vi "Get All Process Names.vi"(11 "?":T9 {"Main Config"."PR Module Configs"."Settings"."PID 2 Parameters"."output range"."output low" format="%.2f"; "Main Config"."PR Module Configs"."Settings"."PID 2 Parameters"."output range"."output high" min=0.0 max=100.0 format="%.2f"; "Main Config"."PR Module Configs"."Settings"."PID 2 Parameters"."PID gains"."derivative time (Td, min)" format="%.3f"; "Main Config"."PR Module Configs"."Settings"."PID 2 Parameters"."PID gains"."integral time (Ti, min)" format="%.3f"; "Main Config"."PR Module Configs"."Settings"."PID 2 Parameters"."PID gains"."proportional gain (Kc)" format="%.3f"; "Main Config"."Steps"."Control" items=["Pump %", "Setpoint"]; "Main Config"."TCU Module Configs"."Settings"."Huber Unistat 410 Settings"."Address" min=0 max=99 format="%02.0f"; "Main Config"."TCU Module Configs"."Settings"."Julabo FP-50 Settings"."Pump Power" min=0 max=8 step=1; "Main Config"."TCU Module Configs"."Settings"."Lauda Settings"."Pump Power" min=0 max=8 step=1; "Main Config"."Pump Module Configs"."Settings"."ASIA Pump C"."channel" min=0 max=1 step=1; "Main Config"."Pump Module Configs"."Settings"."Masterflex"."Pump Number" min=1.0 max=20.0 step=1.0; "Main Config"."Pump Module Configs"."Settings"."Ismatech"."Pump Number" min=1.0 max=20.0 step=1.0; "Main Config"."Feed Module Configs"."Settings"."output range"."output low" min=0.0 max=100.0 format="%.2f"; "Main Config"."Feed Module Configs"."Settings"."output range"."output high" format="%.2f"; "Main Config"."Feed Module Configs"."Settings"."PID 2 Parameters"."PID gains"."derivative time (Td, min)" format="%.3f"; "Main Config"."Feed Module Configs"."Settings"."PID 2 Parameters"."PID gains"."integral time (Ti, min)" format="%.3f"; "Main Config"."Feed Module Configs"."Settings"."PID 2 Parameters"."PID gains"."proportional gain (Kc)" format="%.3f"; "Main Config"."Feed Module Configs"."Settings"."ASIA Pump C"."channel" min=0 max=1 step=1; "Main Config"."Feed Module Configs"."Settings"."Ismatech"."Pump Number" min=1.0 max=20.0 step=1.0; "Main Config"."Feed Module Configs"."Settings"."Masterflex"."Pump Number" min=1.0 max=20.0 step=1.0}) -> (3 "Module Tags Array Cluster":T6)   [LabVIEW 2018]
uses:
  Drag and Drop/State Cluster.ctl
  Message Queue/Message Cluster.ctl
  Drag and Drop/Thumbnail Cluster.ctl
  Drag and Drop/Object Cluster.ctl
  <vilib>/Utility/miscctls.llb/LVRectTypeDef.ctl
  Drag and Drop/Object Type Enum.ctl
  <vilib>/Utility/miscctls.llb/LVPositionTypeDef.ctl
  Config Module/Controls/Main Config Cluster.ctl
  OPC/OPC Module Config.ctl
  Scale Module Folder/Measure Instrument/State Enum.ctl
  <vilib>/Utility/miscctls.llb/LVPoint32TypeDef.ctl
  OPC/OPC Settings.ctl
  OPC/Variable Data Cluster.ctl
  <vilib>/OPCUA/controls/NodeId.ctl
  <vilib>/OPCUA/controls/OPC UA StatusCode.ctl
  <vilib>/OPCUA/controls/Subscription ID.ctl
  <vilib>/OPCUA/controls/OPC UA Client Refnum.ctl
  <vilib>/OPCUA/controls/Subscription Data Change.ctl
  <vilib>/OPCUA/controls/Data Type.ctl
  Feed Module/Controls/Feed Module Config Cluster.ctl
  Feed Module/Controls/Feed Module Settings Cluster.ctl
  Ismatec ISM 831C/Controls/Ismatech Settings Cluster.ctl
  Masterflex 7550-30/Controls/Settings Cluster.ctl
  Mettler Toledo/Controls/Settings Cluster.ctl
  Bronkhorst M13 Flow Meter/Settings Cluster.ctl
  Measure Instrument/PID 2 Parameters Cluster.ctl
  Measure Instrument/PID Input Enum.ctl
  Measure Instrument/PID 2 Output Enum.ctl
  Tacmina QI/Tacmina QI DAQ Setting.ctl
  KNF Pump/Settings Cluster plus SIMDOS.ctl
  ASIA Pump/Pump Settings.ctl
  VICI M50 Party Mode/Settings Cluster.ctl
  FLOM Pump/Settings Cluster.ctl
  SSI PR Class/SSI PR or LD Settings Cluster.ctl
  Masterflex 75211/Masterflex 75211 DAQ Setting.ctl
  SSI PR Class/SSI P40 Settings Cluster.ctl
  TT Module/Controls/TT Module Config Cluster.ctl
  Tag VIs/Numeric Alarm Settings Cluster.ctl
  Acquisition/Hardware Configuration.ctl
  Acquisition/Task Cluster.ctl
  PT Module/Controls/PT Module Config Cluster.ctl
  Scale Module Folder/Feed Module/Controls/Scale Module Config Cluster.ctl
  Scale Module Folder/Feed Module/Controls/Scale Module Settings Cluster.ctl
  Pump Module Folder/Pump Module Config Cluster.ctl
  Pump Module Folder/Pump Module Settings Cluster.ctl
  LabJack Module/Controls/U3 Module Config Cluster.ctl
  Decoration Module/Decoration Module Config Cluster.ctl
  Flow Module Folder/Feed Module/Controls/Flow Module Config Cluster.ctl
  Flow Module Folder/Feed Module/Controls/Flow Module Settings Cluster.ctl
  TCU Module/TCU Module Folder/TCU Module Config Cluster.ctl
  TCU Module/TCU Module Folder/TCU Module Settings Cluster.ctl
  TCU Module/TCU Module Folder/Measure Instrument/Output Devices.ctl
  Huber TCU/Huber Settings.ctl
  Lauda Integral XT-150 TCU/Lauda Settings.ctl
  Julabo Type 1 TCU/Julabo Type 1 TCU Folder/Julabo FP-50 Settings.ctl
  Huber Unistat 410 TCU/Huber Unistat 410 RS485 Settings.ctl
  D-O Module Folder/Not Sure Where this is Used.ctl
  Sequencing/Squence Control.ctl
  D-O Module Folder/D-O Module Config Cluster.ctl
  D-O Module Folder/Valve Clusters.ctl
  D-O Module Folder/D-O Module Settings Cluster.ctl
  D-O Module Folder/D-O Device Settings Cluster.ctl
  VICI Electronic Actuator/VICI Electronic Actuator Settings.ctl
  Pressure Regulator Control Module/Pressure Regulator/Controls/4-20mA Module Config Cluster.ctl
  Pressure Regulator Control Module/Pressure Regulator/Controls/4-20mA Module Settings Cluster.ctl
  Pressure Transmitter/Pressure Transmitter Device Settings.ctl
  Pressure Reg Module/Pressure Regulator Device Settings.ctl
  Feed Module/Controls/Feed Module Tag Names Cluster.ctl
  Pump Module Folder/Pump Module Tag Names Cluster.ctl
  Bronkhorst M14 Flow Meter/Tag Cluster.ctl
  TCU Module/TCU Module Folder/TCU Module Tag Names Cluster.ctl
  Pressure Regulator Control Module/Pressure Regulator/Controls/4-20mA Module Tag Names Cluster.ctl
  Message Queue/Message Queue.lvlib
  TT Module/TT Module.lvlib
  Masterflex 7550-30/Masterflex 7550-30.lvlib
  Ismatec ISM 831C/Ismatec ISM 831C.lvlib
  Tacmina QI/Tacmina QI.lvlib
  KNF Pump/KNF SIMDOS.lvlib
  VICI M50 Party Mode/VICI M6 M50 Party Mode.lvlib
  FLOM Pump/FLOM Pump.lvlib
  ASIA Pump.lvlib
  Mettler Toledo/Mettler Toledo.lvlib
  Bronkhorst M13 Flow Meter/Bronkhorst M13 Flow Meter.lvlib
  SSI PR Class/SSI PR or LD Pump.lvlib
  Feed Module/Feed Module.lvlib
  DAQ/DAQ.lvlib
  PT Module/PT Module.lvlib
  Scale Module Folder/Scale Module.lvlib
  Pump Module Folder/Pump Module.lvlib
  LabJack Module/U3 Module.lvlib
  Flow Module Folder/Flow Module.lvlib
  Huber TCU/Huber Ministat 230 TCU.lvlib
  Lauda Integral XT-150 TCU/Lauda TCU.lvlib
  Julabo Type 1 TCU/Julabo Type 1 TCU Folder/Julabo Type FP-50 TCU.lvlib
  TCU Module/TCU Module Folder/TCU Module.lvlib
  Sequencing/Sequencing Library.lvlib
  D-O Module Folder/D-O Module.lvlib
  Pressure Transmitter/Pressure Transmitter Library.lvlib
  Pressure Reg Module/Pressure Regulator Library.lvlib
  Pressure Regulator Control Module/Pressure Regulator/4-20mA Module.lvlib
  OPC/OPC UA.lvlib
  Scale Module Folder/Measure Instrument/Scale Module Engine.lvlib
  Config Module/Config Module.lvlib
  Drag and Drop/Drag and Drop.lvlib
  D-O Module Folder/DIO Valve/VICI Electronic Actuator.lvlib
  Masterflex 75211/Masterflex 75211.lvlib
  SSI PR Class/SSI P40 Pump.lvlib
  Huber Unistat 410 TCU/Huber Unistat 410 TCU.lvlib
panel:
  out "OPC Array":T7(array[cluster])
  out "PR Array":T5[](array[typedef])
  out "TCU Array":T4[](array[typedef])
  out "Flow Array":T3[](array[typedef])
  out "Pump Array":T2[](array[typedef])
  out "Scale Array":T8(array[cluster])
  out "DAQ Array":string[](array[string])
  out "Feed Module Array":T1[](array[typedef])
  out "output array":string[](array[string])
  out "appended array":string[][](array[string])
  # "Instrument Settings"
  # "Instrument Settings"
  # "Output Instruments"
  # "Flow Meter Settings"
  # "Output Instruments"
  # "Scale Settings"
  # "Output Instruments"
  # "Input Instruments"
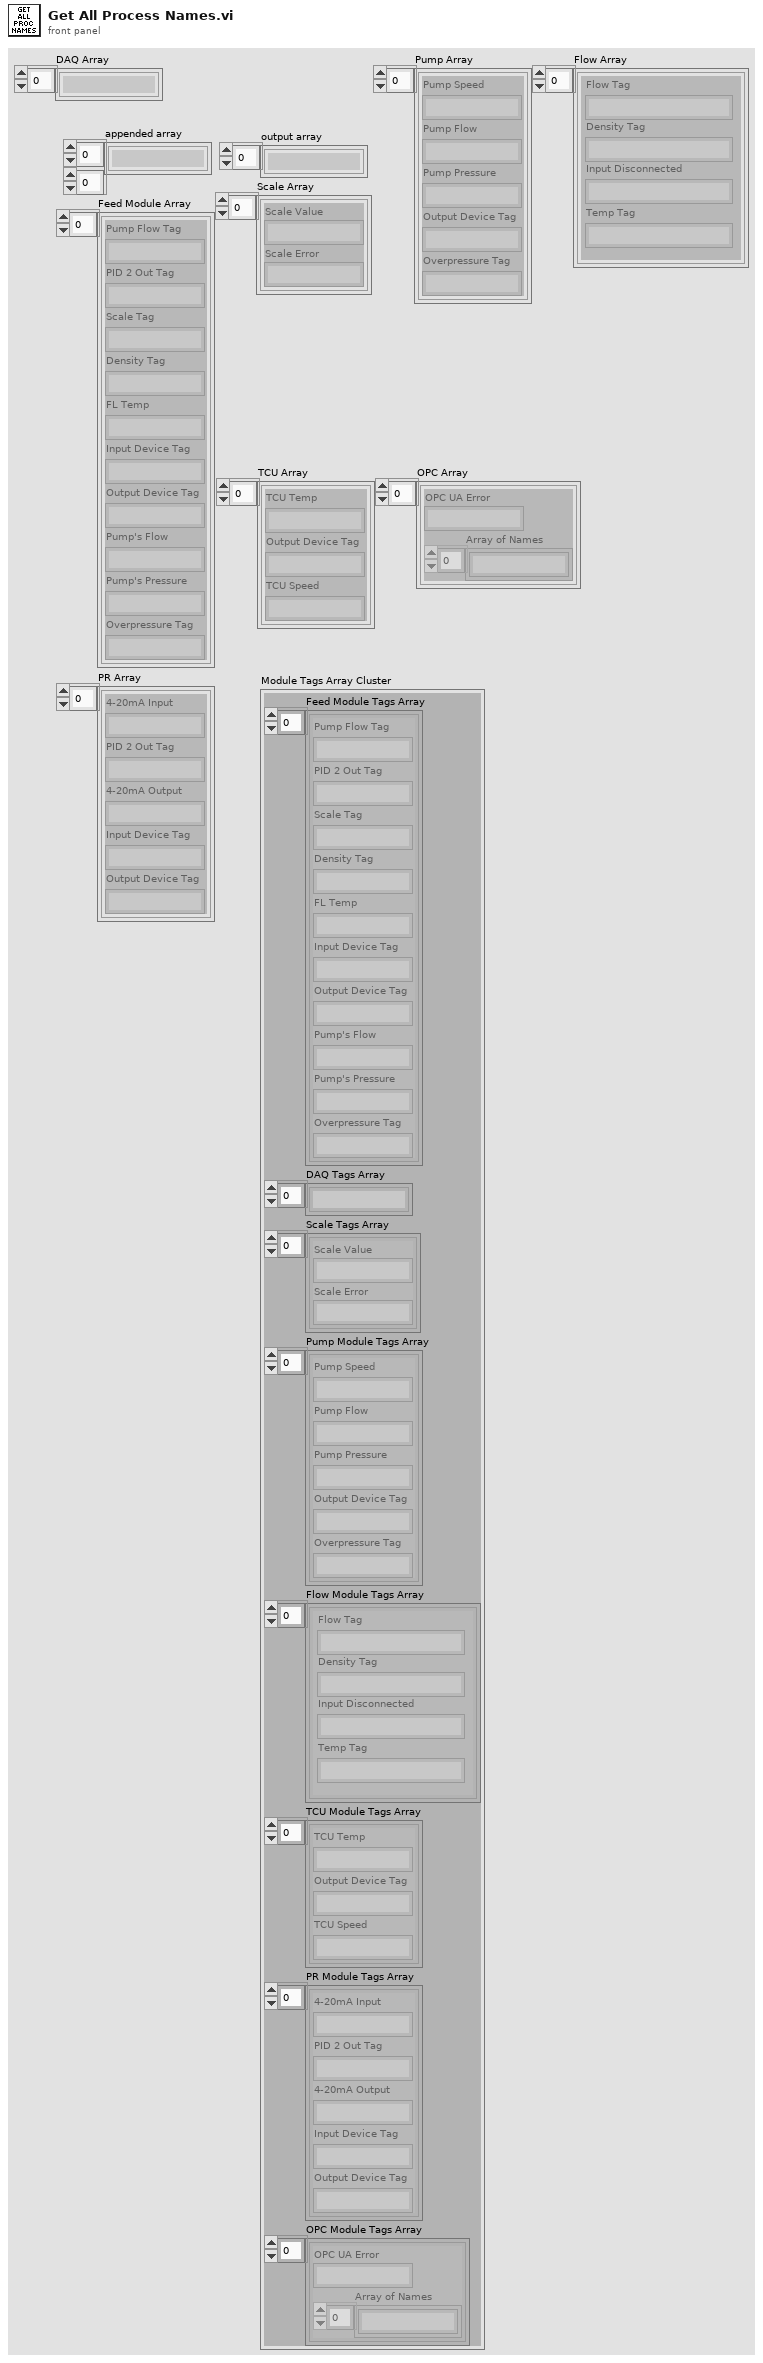
[diagram p1: front panel]
types:
  T1 = typedef "Feed Module.lvlib/Feed Module Tag Names Cluster.ctl" = cluster{"Pump Flow Tag":string, "PID 2 Out Tag":string, "Scale Tag":string, "Density Tag":string, "FL Temp":string, "Input Device Tag":string, "Output Device Tag":string, "Pump's Flow":string, "Pump's Pressure":string, "Overpressure Tag":string}
  T2 = typedef "Pump Module.lvlib/Pump Module Tag Names Cluster.ctl" = cluster{"Pump Speed":string, "Pump Flow":string, "Pump Pressure":string, "Output Device Tag":string, "Overpressure Tag":string}
  T3 = typedef "Flow Module.lvlib/Tag Cluster.ctl" = cluster{"Flow Tag":string, "Input Disconnected":string, "Density Tag":string, "Temp Tag":string}
  T4 = typedef "TCU Module.lvlib/TCU Module Tag Names Cluster.ctl" = cluster{"TCU Temp":string, "Output Device Tag":string, "TCU Speed":string}
  T5 = typedef "4-20mA Module.lvlib/4-20mA Module Tag Names Cluster.ctl" = cluster{"4-20mA Input":string, "PID 2 Out Tag":string, "4-20mA Output":string, "Input Device Tag":string, "Output Device Tag":string}
  T6 = cluster{"Feed Module Tags Array":T1[], "DAQ Tags Array":string[], "Scale Tags Array":cluster{"Scale Value":string, "Scale Error":string}[], "Pump Module Tags Array":T2[], "Flow Module Tags Array":T3[], "TCU Module Tags Array":T4[], "PR Module Tags Array":T5[], "OPC Module Tags Array":cluster{"OPC UA Error":string, "Array of Names":string[]}[]}
  T7 = cluster{"OPC UA Error":string, "Array of Names":string[]}[]
  T8 = cluster{"Scale Value":string, "Scale Error":string}[]
  T9 = typedef "Drag and Drop.lvlib/State Cluster.ctl" = cluster{"VI refs":refnum<vi>[], "Queues":refnum<queue>[], "[Thumbnails]":T10[], "Drag Object Idx":i32, "[Objects]":T11[], "Active Object":i32, "Drop Offset":T14, "Process Name":string, "Main Config":T15, "Campaign Filepath":path, "Config Changed?":bool}
  T10 = typedef "Thumbnail Cluster.ctl" = cluster{"Path":path, "Rectangle":cluster{"left":i16, "top":i16, "right":i16, "bottom":i16}}
  T11 = typedef "Object Cluster.ctl" = cluster{"BMP Path":path, "Anchor Position":cluster{"X":i32, "Y":i32}, "Hot Spot":T12, "Type":T13, "Parameters":variant}
  T12 = typedef "LVRectTypeDef.ctl" = cluster{"Left":i16, "Top":i16, "Right":i16, "Bottom":i16}
  T13 = typedef "Object Type Enum.ctl" = enum16{"Icon", "Line", "Text", "Feed Module"}
  T14 = typedef "LVPositionTypeDef.ctl" = cluster{"Left":i32, "Top":i32}
  T15 = typedef "Config Module.lvlib/Main Config Cluster.ctl" = cluster{"Notebook":string, "Page":string, "OPC Module Configs":T16[], "Feed Module Configs":T25[], "Log File Path":path, "TT Module Configs":T42[], "DAQ Config":T44, "PT Module Configs":T46[], "Scale Module Configs":T47[], "Pump Module Configs":T49[], "U3 Module Configs":T51[], "Decoration Module Configs":T52[], "Flow Module Configs":T53[], "TCU Module Configs":T55[], "Steps":T62, "Abort":bool, "DO Module Configs":T64[], "PR Module Configs":T69[], "Cycle Period":dbl}
  T16 = typedef "OPC UA.lvlib/OPC Module Config.ctl" = cluster{"State":T17, "GUID":string, "Drop Coords":T18, "Configuration":T19, "First Iteration":bool, "Data":cluster{"Object Name":string, "Variable Array":T20[]}[], "Process Name":string, "Load Count":i32, "Log Started":bool, "subscription ID out":T23, "OPC UA client refnum out":T24, "Event Registration Refnum":refnum<event-registration>, "Start Time":timestamp, "Current Time":timestamp}
  T17 = typedef "Scale Module.lvlib/Scale Module Engine.lvlib/State Enum.ctl" = enum16{"Measuring", "Idle"}
  T18 = typedef "LVPoint32TypeDef.ctl" = cluster{"Horizontal":i32, "Vertical":i32}
  T19 = typedef "OPC UA.lvlib/OPC Settings.ctl" = cluster{"Cycle Period":dbl, "server endpoint URL":string, "security policy":cluster{"message mode":enum16{"None", "Sign", "Sign and Encrypt"}, "security":enum16{"Basic256", "Basic128Rsa15"}}, "Trust Any Server":bool}
  T20 = typedef "OPC UA.lvlib/Variable Data Cluster.ctl" = cluster{"node ID":T21, "browse name":string, "status":T22, "timestamp":timestamp, "value ":variant}
  T21 = typedef "NodeId.ctl" = string
  T22 = typedef "OPC UA StatusCode.ctl" = u32
  T23 = typedef "Subscription ID.ctl" = u32
  T24 = typedef "OPC UA Client Refnum.ctl" = refnum<k21>
  T25 = typedef "Feed Module.lvlib/Feed Module Config Cluster.ctl" = cluster{"GUID":string, "Drop Coords":T18, "Process Name":string, "Queue Name":string, "Settings":T26, "Settings Load Count":i32, "OP Load Count":i32}
  T26 = typedef "Feed Module.lvlib/Feed Module Settings Cluster.ctl" = cluster{"Cycle Period":dbl, "Ismatech":T27, "Masterflex":T28, "Mettler":T29, "Bronkhorst M13 Flow Meter":T30, "PID 2 Parameters":T31, "Manual Entry":dbl, "Auto?":bool, "output range":cluster{"output high":dbl, "output low":dbl}, "Bronkhorst M14":T29, "Tacmina Settings":T34, "KNF SIMDOS Settings":T35, "ASIA Pump C":T36, "VICI Settings":T37, "FLOM Settings":T38, "SSI PR/LD Settings":T39, "Masterflex 75211 Settings":T40, "SSI P40 Settings":T41}
  T27 = typedef "Ismatec ISM 831C.lvlib/Ismatech Settings Cluster.ctl" = cluster{"VISA resource name":refnum<visa-resource-name>, "Simulated?":bool, "Pump Number":dbl, "Reverse?":bool}
  T28 = typedef "Masterflex 7550-30.lvlib/Settings Cluster.ctl" = cluster{"VISA resource name":refnum<visa-resource-name>, "Simulated?":bool, "Pump Number":dbl, "Reverse?":bool}
  T29 = typedef "Mettler Toledo.lvlib/Settings Cluster.ctl" = cluster{"VISA resource name":refnum<visa-resource-name>, "Simulated?":bool}
  T30 = typedef "Bronkhorst M13 Flow Meter.lvlib/Settings Cluster.ctl" = cluster{"VISA resource name":refnum<visa-resource-name>, "Simulated?":bool}
  T31 = typedef "PID 2 Parameters Cluster.ctl" = cluster{"Input Device":T32, "Output Device":T33, "Setpoint":dbl, "PID gains":cluster{"proportional gain (Kc)":dbl, "integral time (Ti, min)":dbl, "derivative time (Td, min)":dbl}}
  T32 = typedef "PID Input Enum.ctl" = enum16{"Default", "Bronkhorst M13", "Bronkhorst M14", "Scale Rate of Change"}
  T33 = typedef "PID 2 Output Enum.ctl" = enum16{"Default", "Ismatec ISM 831C", "Masterflex 7550-30", "VICI", "Tacmina QI", "KNF SIMDOS", "ASIA Type C", "FLOM UI-22-11", "SSI PR/LD", "SSI P40", "Masterflex 75211-70"}
  T34 = typedef "Tacmina QI.lvlib/Tacmina QI DAQ Setting.ctl" = cluster{"Analog DAQ Task":refnum<k21>, "Digital DAQ Task":refnum<k21>}
  T35 = typedef "KNF SIMDOS.lvlib/Settings Cluster plus SIMDOS.ctl" = cluster{"VISA resource name":refnum<visa-resource-name>, "Simulated?":bool}
  T36 = typedef "ASIA Pump.lvlib/Pump Settings.ctl" = cluster{"ASIA Pump #":i32, "channel":i32, "Simulated":bool}
  T37 = typedef "VICI M6 M50 Party Mode.lvlib/Settings Cluster.ctl" = cluster{"VISA resource name":refnum<visa-resource-name>, "Simulated?":bool, "Pump Letter":string, "Reverse?":bool}
  T38 = typedef "FLOM Pump.lvlib/Settings Cluster.ctl" = cluster{"VISA resource name":refnum<visa-resource-name>, "Simulated?":bool, "Pump Number":dbl}
  T39 = typedef "SSI PR or LD Pump.lvlib/SSI PR or LD Settings Cluster.ctl" = cluster{"VISA resource name":refnum<visa-resource-name>, "Simulated?":bool}
  T40 = typedef "Masterflex 75211.lvlib/Masterflex 75211 DAQ Setting.ctl" = cluster{"Analog DAQ Task":refnum<k21>, "Digital DAQ Task":refnum<k21>}
  T41 = typedef "SSI P40 Pump.lvlib/SSI P40 Settings Cluster.ctl" = cluster{"VISA resource name":refnum<visa-resource-name>, "Simulated?":bool}
  T42 = typedef "TT Module.lvlib/TT Module Config Cluster.ctl" = cluster{"GUID":string, "Drop Coords":T18, "Input Channel Tag Name ":string, "Process Name":string, "Queue Name":string, "Input Channel Numeric Alarm Settings":T43[]}
  T43 = typedef "Numeric Alarm Settings Cluster.ctl" = cluster{"enable? (F)":bool, "name":string, "alarm type":enum16{"HI_HI", "HI", "LO", "LO_LO"}, "level/change":dbl, "deadband/time":dbl, "alarm delay":dbl, "priority":u32, "ack type":enum16{"Auto", "User", "None", "Each Occurrence"}, "area":string, "description":string, "log? (T)":bool}
  T44 = typedef "DAQ.lvlib/Hardware Configuration.ctl" = cluster{"Tasks":T45[]}
  T45 = typedef "Task Cluster.ctl" = cluster{"DAQmx Task":refnum<k21>, "Read-Write Radio":enum32{"Read", "Write"}}
  T46 = typedef "PT Module.lvlib/PT Module Config Cluster.ctl" = cluster{"GUID":string, "Drop Coords":T18, "Input Channel Tag Name ":string, "Process Name":string, "Queue Name":string, "Input Channel Numeric Alarm Settings":T43[]}
  T47 = typedef "Scale Module.lvlib/Scale Module Config Cluster.ctl" = cluster{"GUID":string, "Drop Coords":T18, "Process Name":string, "Queue Name":string, "Settings":T48, "Load Count":i32}
  T48 = typedef "Scale Module.lvlib/Scale Module Settings Cluster.ctl" = cluster{"Cycle Period":dbl, "Mettler":T29, "Scale Type":string}
  T49 = typedef "Pump Module.lvlib/Pump Module Config Cluster.ctl" = cluster{"GUID":string, "Drop Coords":T18, "Process Name":string, "Queue Name":string, "Settings":T50, "Load Count":i32}
  T50 = typedef "Pump Module.lvlib/Pump Module Settings Cluster.ctl" = cluster{"Cycle Period":dbl, "Manual Entry":dbl, "Output Device":T33, "Ismatech":T27, "Masterflex":T28, "VICI Settings":T37, "Tacmina Settings":T34, "KNF SIMDOS Settings":T35, "ASIA Pump C":T36, "FLOM Settings":T38, "SSI PR/LD Settings":T39, "SSI P40 Settings":T39, "Masterflex 75211 Settings":T40, "Pump Calibration File":path, "Calibration Slope":dbl, "Calibration Y Intercept":dbl, "Pump Cal Enum":u16}
  T51 = typedef "U3 Module.lvlib/U3 Module Config Cluster.ctl" = cluster{"GUID":string, "Drop Coords":T18, "AI Channel Number":enum16{"Default", "AI0", "AI1", "AI2", "AI3", "AI4", "AI5", "AI6", "AI7"}, "Process Name":string, "Queue Name":string, "Input Channel Numeric Alarm Settings":T43[]}
  T52 = typedef "Decoration Module Config Cluster.ctl" = cluster{"GUID":string, "Drop Coords":T18, "Decoration Filepath":path}
  T53 = typedef "Flow Module.lvlib/Flow Module Config Cluster.ctl" = cluster{"GUID":string, "Drop Coords":T18, "Process Name":string, "Queue Name":string, "Settings":T54, "Load Count":i32}
  T54 = typedef "Flow Module.lvlib/Flow Module Settings Cluster.ctl" = cluster{"Cycle Period":dbl, "Bronkhorst M13":T29, "Flow Meter Type":string, "Bronkhorst M14":T29}
  T55 = typedef "TCU Module.lvlib/TCU Module Config Cluster.ctl" = cluster{"GUID":string, "Drop Coords":T18, "Process Name":string, "Queue Name":string, "Settings":T56, "Load Count":i32, "Power Level Changed":bool}
  T56 = typedef "TCU Module.lvlib/TCU Module Settings Cluster.ctl" = cluster{"Cycle Period":dbl, "Setpoint Entry":dbl, "Output Device":T57, "Huber Ministat 230 Settings":T58, "Lauda Settings":T59, "Julabo FP-50 Settings":T60, "Internal Control?":bool, "Huber Unistat 410 Settings":T61}
  T57 = typedef "Output Devices.ctl" = enum16{"Default", "Huber Ministat 230", "Huber Unistat 410", "Lauda XT-150", "Julabo FP-50"}
  T58 = typedef "Huber Ministat 230 TCU.lvlib/Huber Settings.ctl" = cluster{"VISA resource name":refnum<visa-resource-name>, "Simulated?":bool}
  T59 = typedef "Lauda TCU.lvlib/Lauda Settings.ctl" = cluster{"VISA resource name":refnum<visa-resource-name>, "Simulated?":bool, "Pump Power":i32}
  T60 = typedef "Julabo Type FP-50 TCU.lvlib/Julabo FP-50 Settings.ctl" = cluster{"VISA resource name":refnum<visa-resource-name>, "Simulated?":bool, "Pump Power":i32}
  T61 = typedef "Huber Unistat 410 TCU.lvlib/Huber Unistat 410 RS485 Settings.ctl" = cluster{"VISA resource name":refnum<visa-resource-name>, "Address":i8, "Simulated?":bool}
  T62 = typedef "Not Sure Where this is Used.ctl" = T63[]
  T63 = typedef "Sequencing Library.lvlib/Squence Control.ctl" = cluster{"Module":string, "Control":u16, "Value":dbl, "Wait (sec)":dbl}
  T64 = typedef "D-O Module.lvlib/D-O Module Config Cluster.ctl" = cluster{"GUID":string, "Drop Coords":T18, "Process Name":string, "Queue Name":string, "Settings":T65, "Load Count":i32}
  T65 = typedef "D-O Module.lvlib/Valve Clusters.ctl" = cluster{"Valve Settings":T66, "Valve Type":enum16{"Default", "Digital Output Valve", "VICI Electronic Actuator"}, "Time On (Sec)":dbl, "Time Off (Sec)":dbl, "Run?":bool}
  T66 = typedef "D-O Module.lvlib/D-O Module Settings Cluster.ctl" = cluster{"D-O Settings":T67, "VICI Electronic Actuator":T68}
  T67 = typedef "D-O Module.lvlib/D-O Device Settings Cluster.ctl" = cluster{"DAQmx Task Name":refnum<k21>, "Output Channel":u16, "Output Channel Names":string[]}
  T68 = typedef "VICI Electronic Actuator.lvlib/VICI Electronic Actuator Settings.ctl" = cluster{"VISA resource name":refnum<visa-resource-name>, "Mode":enum16{"Two Positions With Stops", "Two Positions Without Stops", "Mutiposition"}, "Simulated":bool}
  T69 = typedef "4-20mA Module.lvlib/4-20mA Module Config Cluster.ctl" = cluster{"GUID":string, "Drop Coords":T18, "Process Name":string, "Queue Name":string, "Settings":T70, "Settings Load Count":i32}
  T70 = typedef "4-20mA Module.lvlib/4-20mA Module Settings Cluster.ctl" = cluster{"Cycle Period":dbl, "PID 2 Parameters":cluster{"Input Device":enum16{"Default", "4-20mA"}, "Output Device":enum16{"Default", "Equilibar Pressure Reg", "Flow Regulator"}, "Setpoint":dbl, "PID gains":cluster{"proportional gain (Kc)":dbl, "integral time (Ti, min)":dbl, "derivative time (Td, min)":dbl}, "output range":cluster{"output low":dbl, "output high":dbl}}, "Manual Entry":dbl, "Auto?":bool, "4-20mA Input Settings":T71, "4-20mA Out Settings":T72, "Input Channel Tag Name ":string}
  T71 = typedef "Pressure Transmitter Library.lvlib/Pressure Transmitter Device Settings.ctl" = cluster{"Input Channel ":u16}
  T72 = typedef "Pressure Regulator Library.lvlib/Pressure Regulator Device Settings.ctl" = cluster{"Output DAQ Task":refnum<k21>}
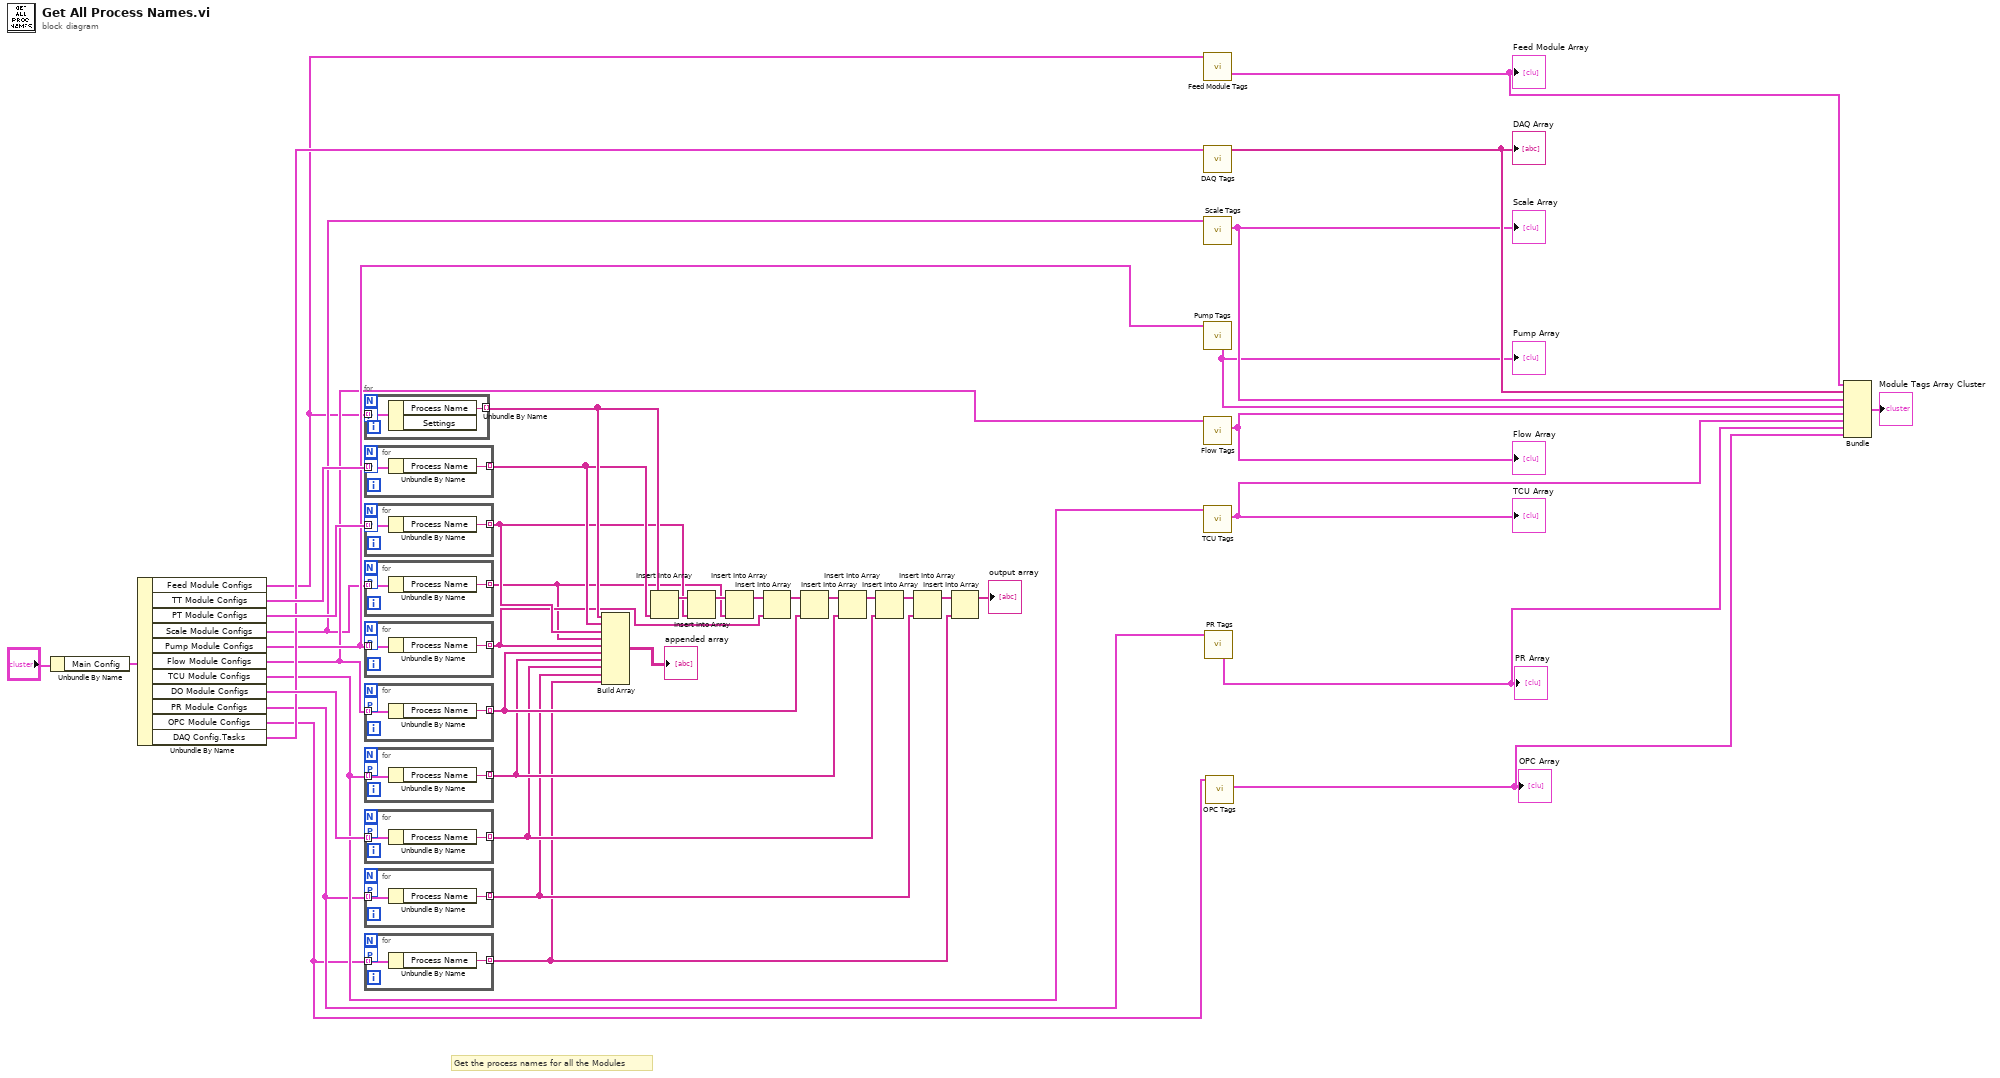
[diagram p0: block diagram]
diagram:
  # "Get the process names for all the Modules"
  n1 = Unbundle By Name("?") -> ("Main Config"=w42:T15)
  n2 = Unbundle By Name(w42) -> ("Feed Module Configs"=w2:T25[], "TT Module Configs"=w40:T42[], "PT Module Configs"=w39:T46[], "Scale Module Configs"=w14:T47[], "Pump Module Configs"=w16:T49[], "Flow Module Configs"=w15:T53[], "TCU Module Configs"=w13:T55[], "DO Module Configs"=w38:T64[], "PR Module Configs"=w12:T69[], "OPC Module Configs"=w11:T16[], "DAQ Config.Tasks"=w18:T45[])
  n3 = for {
    tunnel: w2 -> [w44] mode=indexing
    tunnel: [w43] -> w36 mode=indexing
    workers-P: _ -> [_]
    n4 = Unbundle By Name(w44) -> ("Process Name"=w43:string)  [unwired: 1 out]
  }
  n5 = for {
    tunnel: w40 -> [w46] mode=indexing
    tunnel: [w45] -> w35 mode=indexing
    workers-P: _ -> [_]
    n6 = Unbundle By Name(w46) -> ("Process Name"=w45:string)
  }
  n7 = for {
    tunnel: w39 -> [w48] mode=indexing
    tunnel: [w47] -> w33 mode=indexing
    workers-P: _ -> [_]
    n8 = Unbundle By Name(w48) -> ("Process Name"=w47:string)
  }
  n9 = for {
    tunnel: w14 -> [w50] mode=indexing
    tunnel: [w49] -> w17 mode=indexing
    workers-P: _ -> [_]
    n10 = Unbundle By Name(w50) -> ("Process Name"=w49:string)
  }
  n11 = for {
    tunnel: w16 -> [w52] mode=indexing
    tunnel: [w51] -> w30 mode=indexing
    workers-P: _ -> [_]
    n12 = Unbundle By Name(w52) -> ("Process Name"=w51:string)
  }
  n13 = for {
    tunnel: w15 -> [w54] mode=indexing
    tunnel: [w53] -> w28 mode=indexing
    workers-P: _ -> [_]
    n14 = Unbundle By Name(w54) -> ("Process Name"=w53:string)
  }
  n15 = for {
    tunnel: w13 -> [w56] mode=indexing
    tunnel: [w55] -> w26 mode=indexing
    workers-P: _ -> [_]
    n16 = Unbundle By Name(w56) -> ("Process Name"=w55:string)
  }
  n17 = for {
    tunnel: w38 -> [w58] mode=indexing
    tunnel: [w57] -> w24 mode=indexing
    workers-P: _ -> [_]
    n18 = Unbundle By Name(w58) -> ("Process Name"=w57:string)
  }
  n19 = for {
    tunnel: w12 -> [w60] mode=indexing
    tunnel: [w59] -> w22 mode=indexing
    workers-P: _ -> [_]
    n20 = Unbundle By Name(w60) -> ("Process Name"=w59:string)
  }
  n21 = for {
    tunnel: w11 -> [w62] mode=indexing
    tunnel: [w61] -> w20 mode=indexing
    workers-P: _ -> [_]
    n22 = Unbundle By Name(w62) -> ("Process Name"=w61:string)
  }
  n23 = Build Array(w36, w35, w33, w17, w30, w28, w26, w24, w22, w20) -> (→"appended array":string[][])
  n24 = Insert Into Array(array=w36, new element=w35) -> (w34:string[])  [unwired: 1 in]
  n25 = Insert Into Array(array=w34, new element=w33) -> (w32:string[])  [unwired: 1 in]
  n26 = Insert Into Array(array=w32, new element=w17) -> (w31:string[])  [unwired: 1 in]
  n27 = Insert Into Array(array=w31, new element=w30) -> (w29:string[])  [unwired: 1 in]
  n28 = Insert Into Array(array=w29, new element=w28) -> (w27:string[])  [unwired: 1 in]
  n29 = Insert Into Array(array=w27, new element=w26) -> (w25:string[])  [unwired: 1 in]
  n30 = Insert Into Array(array=w25, new element=w24) -> (w23:string[])  [unwired: 1 in]
  n31 = Insert Into Array(array=w23, new element=w22) -> (w21:string[])  [unwired: 1 in]
  n32 = Insert Into Array(array=w21, new element=w20) -> (→"output array":string[])  [unwired: 1 in]
  n33 = call "Feed Module Tags.vi"("Feed Module Configs"=w2) -> ("Feed Module Tags Array"=w10:T1[])  [unwired: 6 in, 8 out]
  "Feed Module Array" <- w10
  n34 = call "DAQ Tags.vi"("Tasks"=w18) -> ("DAQ Tags Array"=w9:string[])  [unwired: 10 in]
  "DAQ Array" <- w9
  n35 = call "Scale Tags.vi"("Scale Module Configs"=w14) -> ("Scale Tags Array"=w8:T8)  [unwired: 8 in, 2 out]
  "Scale Array" <- w8
  n36 = call "Pump Tags.vi"("Pump Module Configs"=w16) -> ("Pump Module Tags Array"=w7:T2[])  [unwired: 7 in, 3 out]
  "Pump Array" <- w7
  n37 = call "Flow Tags.vi"("Flow Module Configs"=w15) -> ("Flow Module Tags Array"=w6:T3[])  [unwired: 7 in, 3 out]
  "Flow Array" <- w6
  n38 = call "TCU Tags.vi"("TCU Module Configs"=w13) -> ("TCU Module Tags Array"=w5:T4[])  [unwired: 7 in, 3 out]
  "TCU Array" <- w5
  n39 = call "PR Tags.vi"("PR Module Configs"=w12) -> ("PR Module Tags Array"=w4:T5[])  [unwired: 6 in, 4 out]
  "PR Array" <- w4
  n40 = call "OPC Tags.vi"("OPC Module Configs"=w11) -> ("OPC Module Tags Array"=w3:T7)  [unwired: 7 in, 3 out]
  "OPC Array" <- w3
  n41 = Bundle("Feed Module Tags Array"=w10, "DAQ Tags Array"=w9, "Scale Tags Array"=w8, "Pump Module Tags Array"=w7, "Flow Module Tags Array"=w6, "TCU Module Tags Array"=w5, "PR Module Tags Array"=w4, "OPC Module Tags Array"=w3) -> (→"Module Tags Array Cluster":T6)  [unwired: 1 in]
